vi "move3.vi"(4 "error in":errorcluster, 7 "file path":path) -> (0 "error out":errorcluster, 3 "new path":path)   [LabVIEW 2010]
panel:
  out "date/time string":string
  out "filenames":string[](array[string])
  # "Удаляет дату из названия."
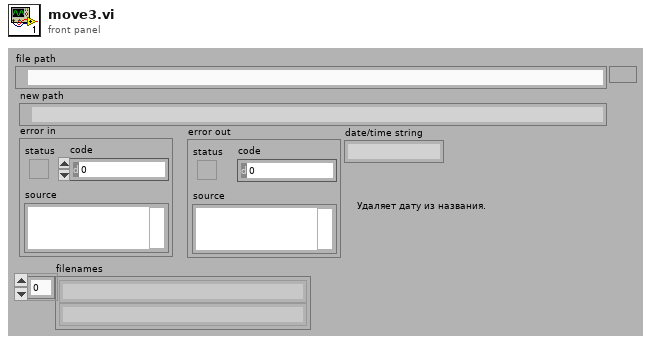
[diagram p1: front panel]
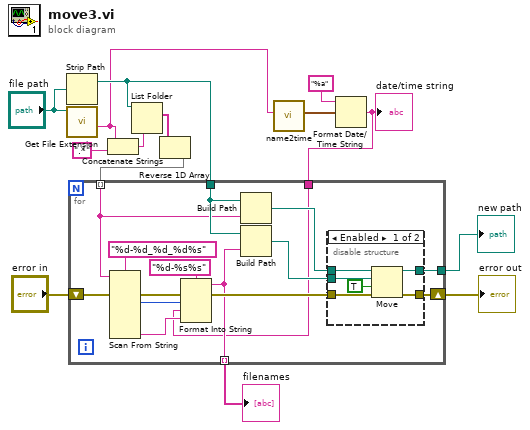
[diagram p0: block diagram]
diagram:
  n1 = Strip Path(path="file path") -> (stripped path=w11:path)  [unwired: 1 out]
  n2 = call <vilib>:"Get File Extension.vi"("file"="file path") -> ("filename without extension"=w4:string)  [unwired: 7 in, 3 out]
  n3 = Concatenate Strings(w4, ".*" ("string")) -> (w9:string)
  n4 = List Folder(path=w11, pattern=w9) -> (filenames=w7:string[])  [unwired: 2 in, 3 out]
  n5 = Reverse 1D Array(array=w7) -> (reversed array=w5:string[])
  n6 = call "name2time.vi"("f_name"=w4) -> ("time stamp"=w3:timestamp)  [unwired: 4 in, 2 out]
  n7 = Format Date/Time String(time format string (%c)="%a", seconds (now)=w3) -> (date/time string=w1:string)  [unwired: 1 in]
  "date/time string" <- w1
  n8 = for {
    tunnel: [w28] -> w13
    tunnel: w5 -> [w18] mode=indexing
    tunnel: w11 -> [w19]
    tunnel: [w21] -> w6 mode=indexing
    shift-right: [w29] -> w14
    shift-left: "error in" -> [w24]
    tunnel: w1 -> [w15]
    n9 = Scan From String(format string="%d-%d_%d_%d%s", input string=w18, error in=w24) -> (error out=w25:errorcluster, output 1=w26:i32, output 5=w16:string)  [unwired: 9 in, 2 out]
    n10 = Format Into String(format string="%d-%s%s", error in=w25, w26, w15, w16) -> (resulting string=w21:string, error out=w23:errorcluster)  [unwired: 1 in]
    n11 = Build Path(base path=w19, name or relative path=w18) -> (appended path=w17:path)
    n12 = Build Path(base path=w19, name or relative path=w21) -> (appended path=w20:path)
    n13 = disable-structure shown="Enabled" {
      disable-tunnel: [w35 w37] -> w29
      disable-tunnel: w23 -> [w34 w37]
      disable-tunnel: [w33 w36] -> w28
      disable-tunnel: w17 -> [w32 _]
      disable-tunnel: w20 -> [w31 w36]
      frame Enabled {
        n14 = Move(source path=w32, error in=w34, 9:TRUE ("overwrite (F)"), 10:w31) -> (error out=w35:errorcluster, 3:w33:path)  [unwired: 1 in, 1 out]
      }
      frame Disabled {
      }
    }
  }
  "error out" <- w14
  "new path" <- w13
  "filenames" <- w6
